vi "getTopThree.vi"(8 "error in (no error)":errorcluster, 11 "ElfHeap in":refnum<class "ElfHeap.lvclass">) -> (0 "error out":errorcluster, 2 "Sum Top Three Carried Calories":dbl)   [LabVIEW 2017, in "ElfHeap.lvclass"]
uses:
  ElfHeap.lvclass
  Elf/Elf.lvclass/Elf.ctl
  Elf/Elf.lvclass
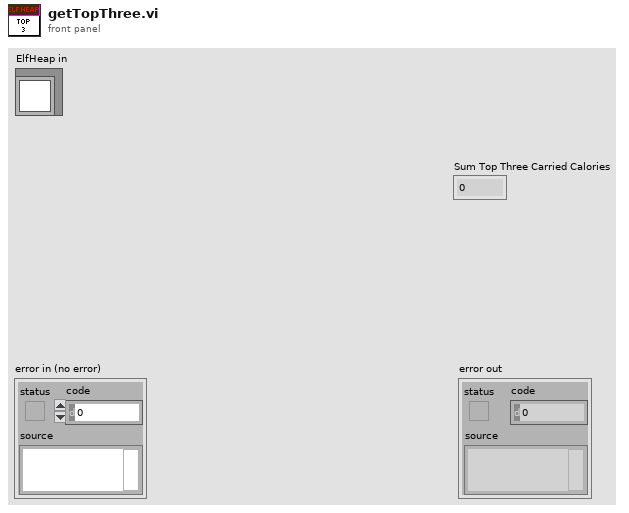
[diagram p1: front panel]
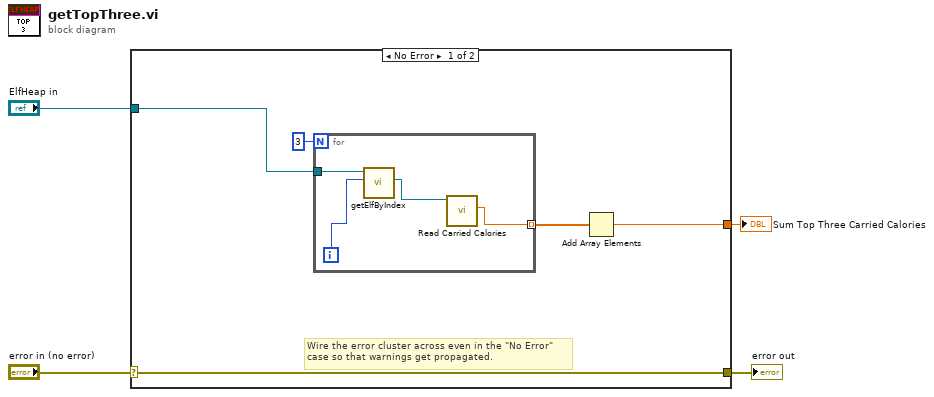
[diagram p0: block diagram]
diagram:
  n1 = case shown="No Error" "error in (no error)" {
    selector: "error in (no error)" -> [w9 w14]
    tunnel: [w9 w14] -> w3
    tunnel: "ElfHeap in" -> [w8 _]
    tunnel: [w5 _] -> w1
    frame No Error {
      # "Wire the error cluster across even in the \"No Error\"\ncase so that warnings get propagated."
      n2 = for {
        N: 3 -> [_]
        tunnel: w8 -> [w12]
        tunnel: [w10] -> w6 mode=indexing
        i -> [w11]
        n3 = call-dynamic "getElfByIndex.vi"("Index"=w11, "ElfHeap in"=w12) -> ("Elf"=w13:refnum<class "Elf.lvclass">)  [unwired: 8 in, 1 out]
        n4 = call "Read Carried Calories.vi"("Elf in"=w13) -> ("Carried Calories"=w10:dbl)  [unwired: 8 in, 2 out]
      }
      n5 = Add Array Elements(numeric array=w6) -> (sum=w5:dbl)
    }
    frame Error {
    }
  }
  "error out" <- w3
  "Sum Top Three Carried Calories" <- w1
